vi "extended_av.vi"(1 "tango data type":T2=enum."STRING_SPE", 2 "num_data":u8[](array[numeric]), 3 "dim. y":i32, 4 "dim. x":i32, 5 "attribute name":string, 6 "device name":string) -> ()   [LabVIEW 2014, in "tango.lvlib"]
uses:
  tango.lvlib
  Common VIs/Typedefs/_AttributeDataType_t.ctl
panel:
  out "extended attribute value":T1
  in  "str_data":string[](array[string])
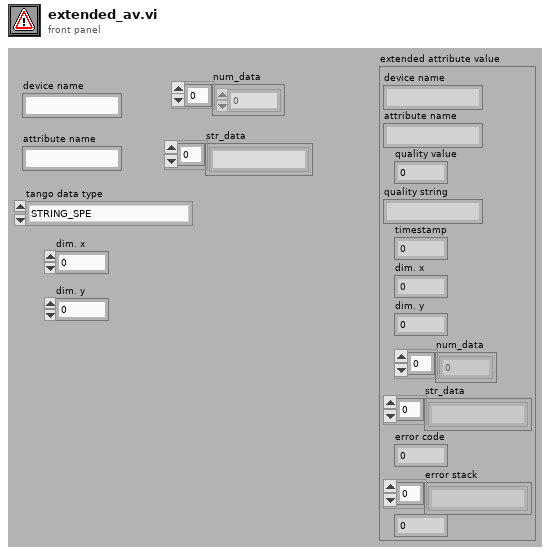
[diagram p1: front panel]
types:
  T1 = cluster{"device name":string, "attribute name":string, "quality value":i16, "quality string":string, "timestamp":dbl, "dim. x":i32, "dim. y":i32, "num_data":u8[], "str_data":string[], "error code":i32, "error stack":string[], u16}
  T2 = typedef "tango.lvlib/_AttributeDataType_t.ctl" = enum16{"STATE_SCA", "STATE_SPE", "STATE_IMG", "STRING_SCA", "STRING_SPE", "STRING_IMG", "BOOL_SCA", "BOOL_SPE", "BOOL_IMG", "UCHAR_SCA", "UCHAR_SPE", "UCHAR_IMG", "SHORT_SCA", "SHORT_SPE", "SHORT_IMG", "USHORT_SCA", "USHORT_SPE", "USHORT_IMG", "LONG_SCA", "LONG_SPE", "LONG_IMG", "ULONG_SCA", "ULONG_SPE", "ULONG_IMG", "LONG64_SCA", "LONG64_SPE", "LONG64_IMG", "ULONG64_SCA", "ULONG64_SPE", "ULONG64_IMG", "FLOAT_SCA", "FLOAT_SPE", "FLOAT_IMG", "DOUBLE_SCA", "DOUBLE_SPE", "DOUBLE_IMG", "UNKNOWN_DATA_TYPE"}
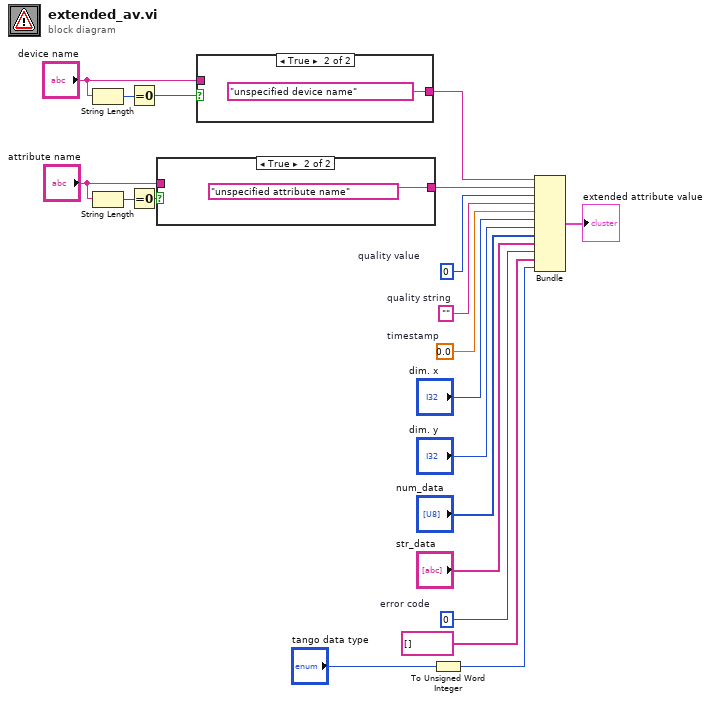
[diagram p0: block diagram]
diagram:
  w4 = 0  # error code
  w17 = 0.0  # timestamp
  w16 = ""  # quality string
  w15 = i16 0  # quality value
  n1 = String Length(string="device name") -> (length=w14:i32)
  n2 = String Length(string="attribute name") -> (length=w10:i32)
  n3 = Equal To 0?(x=w14) -> (x = 0?=w13:bool)
  n4 = Equal To 0?(x=w10) -> (x = 0?=w9:bool)
  n5 = case shown="True" w9 {
    tunnel: "attribute name" -> [w21 _]
    tunnel: [w21 "unspecified attribute name" ("attribute name")] -> w7
    frame False {
    }
    frame True {
    }
  }
  n6 = case shown="True" w13 {
    tunnel: "device name" -> [w23 _]
    tunnel: [w23 "unspecified device name" ("device name")] -> w11
    frame False {
    }
    frame True {
    }
  }
  n7 = To Unsigned Word Integer(number="tango data type") -> (unsigned 16bit integer=w2:u16)
  n8 = Bundle("device name"=w11, "attribute name"=w7, "quality value"=w15, "quality string"=w16, "timestamp"=w17, "dim. x"="dim. x", "dim. y"="dim. y", "num_data"="num_data", "str_data"="str_data", "error code"=w4, "error stack"=string[] [], w2) -> (→"extended attribute value":T1)  [unwired: 1 in]
